vi "Histogram.vi"() -> ()   [LabVIEW 2014]
doc: "Use this template to build a VI to use as a subVI."
uses:
  <vilib>/vision/NI_Vision_Development_Module.lvlib
panel:
  out "Cumulative Histograph":T1(graph)
  out "Histogram Report":T2 {"Standard  Variation" format="%.2f"; "Mean Value" format="%.2f"; "Interval Width" format="%.2f"; "Starting Value" format="%.2f"; "Maximal Value" format="%.2f"; "Minimal Value" format="%.2f"}
  out "Mean Value":sgl format="%.2f"
  out "Standard  Deviation":sgl format="%.2f"
  out "Histograph":T1(graph)
  out "Src":T3(plugin-control)
  # ":: MVi Framework V1.0 ::\nAuthor:Gaoke Yang\nEmail: gaoke.yang@yahoo.com\nWeb: www.mvicontrol.com\nCopyright (C) 2015, MVI Technologies All Rights Reserved"
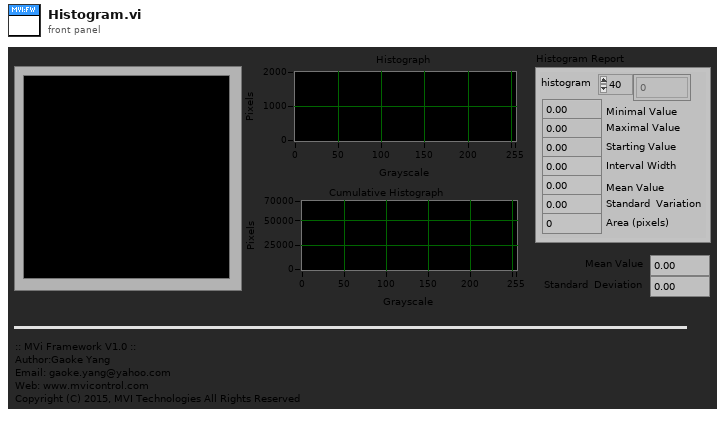
[diagram p1: front panel]
types:
  T1 = cluster{"Starting Value":sgl, "Incremental Value":sgl, "Histogram":u32[]}
  T2 = cluster{"histogram":u32[], "Minimal Value":sgl, "Maximal Value":sgl, "Starting Value":sgl, "Interval Width":sgl, "Mean Value":sgl, "Standard  Variation":sgl, "Area (pixels)":i32}
  T3 = typedef "IMAQ Image.ctl" = refnum<image>
  T4 = typedef "Image Type" = u32
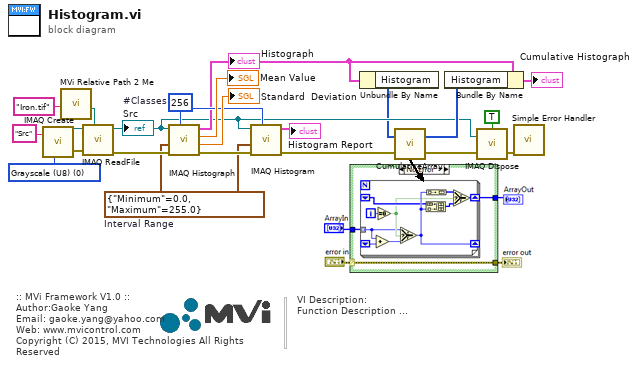
[diagram p0: block diagram]
diagram:
  w9 = 256  # #Classes
  w10 = cluster{"Minimum":sgl, "Maximum":sgl} {"Minimum"=0.0, "Maximum"=255.0}  # Interval Range
  w16 = T4 0 items=["Grayscale (U8)", "Grayscale (I16)", "Grayscale (SGL)", "Complex (CSG)", "RGB (U32)", "HSL (U32)", "RGB (U64)", "Grayscale (U16)"] ("Image Type")
  # "VI Description:\nFunction Description ..."
  # ":: MVi Framework V1.0 ::\nAuthor:Gaoke Yang\nEmail: gaoke.yang@yahoo.com\nWeb: www.mvicontrol.com\nCopyright (C) 2015, MVI Technologies All Rights Reserved"
  n1 = call "IMAQ Create"("Image Name"="Src" ("name or relative path"), "Image Type"=w16) -> ("New Image"=w17:T3, "error out"=w15:errorcluster)  [unwired: 2 in, 1 out]
  n2 = call "MVi Relative Path 2 Me.vi"("Relative Path"="Iron.tif" ("name or relative path")) -> ("Appended Dir"=w18:path)  [unwired: 5 in, 1 out]
  n3 = call "IMAQ ReadFile"("File Path"=w18, "error in (no error)"=w15, "Image"=w17) -> ("error out"=w14:errorcluster, "Image Out"=w2:T3)  [unwired: 4 in, 3 out]
  "Src" <- w2
  n4 = call "IMAQ Histograph"("Number of Classes"=w9, "error in (no error)"=w14, "Interval Range"=w10, "Image"=w2) -> ("error out"=w11:errorcluster, "Standard  Deviation"=→"Standard  Deviation":sgl, "Mean Value"=→"Mean Value":sgl, "Histogram Graph"=w6:T1)  [unwired: 4 in]
  "Histograph" <- w6
  n5 = call "IMAQ Histogram"("Number of Classes"=w9, "error in (no error)"=w11, "Interval Range"=w10, "Image"=w2) -> ("error out"=w5:errorcluster, "Histogram Report"=→"Histogram Report":T2)  [unwired: 6 in]
  n6 = Unbundle By Name(w6) -> ("Histogram"=w1:u32[])
  n7 = call "CumulativeArray.vi"("error in"=w5, "ArrayIn"=w1) -> ("error out"=w3:errorcluster, "ArrayOut"=w7:u32[])
  n8 = Bundle By Name(cluster=w6, "Histogram"=w7) -> (→"Cumulative Histograph":T1)
  n9 = call "IMAQ Dispose"("All Images? (No)"=TRUE, "Image"=w2, "error in (no error)"=w3) -> ("error out"=w19:errorcluster)  [unwired: 3 out]
  n10 = call <vilib>:"Simple Error Handler.vi"("error in (no error)"=w19) -> ()  [unwired: 1 in, 8 out]
